vi "Retrieve Scaling and Convert AO to RawVal.vi"(7 "bypass (F)":bool, 8 "error in (no error)":errorcluster, 9 "EU Value in":dbl, 10 "IOName":string, 11 "DaqDevice dCVT":T1) -> (0 "error out":errorcluster, 1 "Raw Value Out":dbl, 2 "IOName out":string, 3 "DaqDevice dCVT out":T1, 5 "In Range?":bool)   [LabVIEW 2017, in "DAQ.lvclass"]
doc: "Developed by Kevin Thompson\nkevin@thompsonengineering.net\n\nCopyright 2018-2020\nThompson Engineering, LLC"
uses:
  DAQ.lvclass
  <vilib>/TELLC/Dynamic CVT API/TD Dynamic CVT DVR--ref.ctl
  DataTypes/TD AO Channel--cluster.ctl
  DataTypes/TD DataValueConversion--cluster.ctl
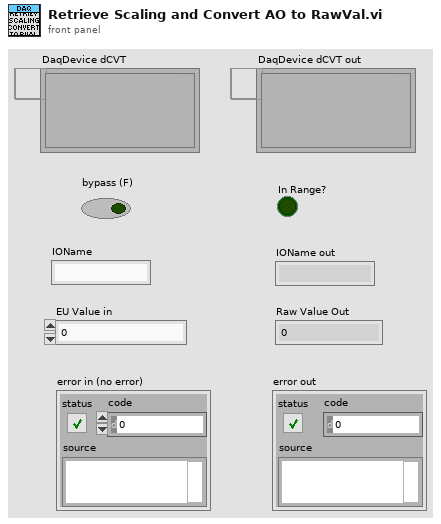
[diagram p1: front panel]
types:
  T1 = typedef "TD Dynamic CVT DVR--ref.ctl" = refnum<data-value>
  T2 = typedef "DAQ.lvclass/TD AO Channel--cluster.ctl" = cluster{"DevName":string, "IOName":string, "IOPath":string, "SchemName":string, "Vmin":dbl, "Vmax":dbl, "Conversion":T3, "DAQmx Task":refnum<k21>}
  T3 = typedef "DAQ.lvclass/TD DataValueConversion--cluster.ctl" = cluster{"MaxSignal":dbl, "MinSignal":dbl, "MaxEngUnit":dbl, "MinEngUnit":dbl, "ScaleOffset":dbl, "negate":bool}
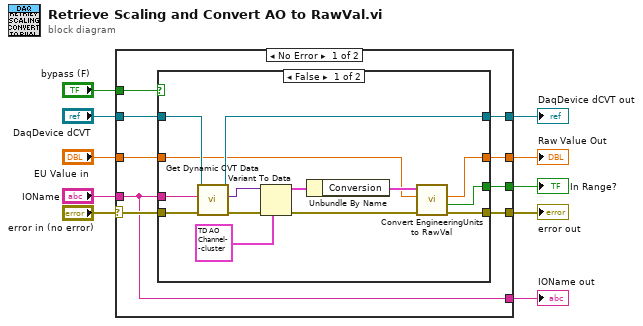
[diagram p0: block diagram]
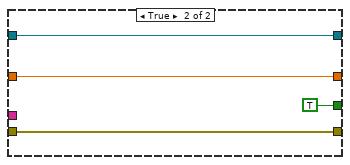
[diagram p2: hidden frame]
diagram:
  n1 = case shown="No Error" "error in (no error)" {
    selector: "error in (no error)" -> [w14 w40]
    tunnel: [w19 w39] -> w10
    tunnel: [w18 w40] -> w9
    tunnel: "IOName" -> [w12 w38]
    tunnel: "DaqDevice dCVT" -> [w17 w41]
    tunnel: [w16 w41] -> w6
    tunnel: "EU Value in" -> [w15 w39]
    tunnel: "bypass (F)" -> [w13 _]
    tunnel: [w12 w38] -> w2
    tunnel: [w11 _] -> w1
    frame No Error {
      n2 = case shown="False" w13 {
        tunnel: [w33 w36] -> w19
        tunnel: [w32 w35] -> w18
        tunnel: w12 -> [w26 _]
        tunnel: w17 -> [w25 w37]
        tunnel: [w24 w37] -> w16
        tunnel: w15 -> [w23 w36]
        tunnel: w14 -> [w22 w35]
        tunnel: [w21 TRUE] -> w11
        frame False {
          n3 = call <vilib>:"Get Dynamic CVT Data.vi"("error in (no error)"=w22, "DataName"=w26, "dCVT DVR"=w25) -> ("error out"=w28:errorcluster, "value"=w27:variant, "dCVT DVR out"=w24:T1)  [unwired: 5 in, 1 out]
          n4 = Variant To Data(error in=w28, type=T2 {"DevName"="", "IOName"="", "IOPath"="", "SchemName"="", "Vmin"=0.0, "Vmax"=0.0, "Conversion"={"MaxSignal"=0.0, "MinSignal"=0.0, "MaxEngUnit"=0.0, "MinEngUnit"=0.0, "ScaleOffset"=0.0, "negate"=FALSE}, "DAQmx Task"=""} ("AO"), Variant=w27) -> (data=w29:T2, error out=w31:errorcluster)
          n5 = Unbundle By Name(w29) -> ("Conversion"=w30:T3)
          n6 = call "Convert EngineeringUnits to RawVal.vi"("error in (no error)"=w31, "Engineering Units In"=w23, "Conversion"=w30) -> ("error out"=w32:errorcluster, "In Range?"=w21:bool, "Raw Value Out"=w33:dbl)  [unwired: 6 in]
        }
        frame True {
        }
      }
    }
    frame Error {
    }
  }
  "Raw Value Out" <- w10
  "error out" <- w9
  "DaqDevice dCVT out" <- w6
  "IOName out" <- w2
  "In Range?" <- w1
